vi "Image UDP Broadcast RT Driver VI.vi"(6 "Device Clock":string, 9 "Device Inputs FIFO":refnum<k33>, 10 "Device Outputs FIFO":refnum<k33>, 11 "Device Reference":T1 format="%.0x") -> ()   [LabVIEW 2012, in "Image UDP Broadcast Custom Device.lvlib"]
uses:
  Shared/Image UDP Broadcast Custom Device.lvlib
  <vilib>/NI Veristand/Custom Device API/Custom Device Item Ref.ctl
  <vilib>/NI Veristand/Custom Device API/Custom Device Channel Type.ctl
  <vilib>/vision/driver/IMAQdx.llb/IMAQdx Acquisition Mode.ctl
  <vilib>/NI Veristand/Custom Device API/Message Response (String).ctl
  <vilib>/NI Veristand/Custom Device API/Message Response (Byte Array).ctl
  <vilib>/vision/driver/IMAQdx.llb/IMAQdx Buffer Number Mode.ctl
  <vilib>/NI Veristand/Custom Device API/Custom Device API.lvlib
  <vilib>/NI Veristand/Custom Device Tools/Custom Device Utility Library/Custom Device Utility Library.lvlib
  <vilib>/vision/driver/NI_Vision_Acquisition_Software.lvlib
  <vilib>/vision/NI_Vision_Development_Module.lvlib
panel:
  in  "Initialization Status Notifier":refnum<notifier>
  in  "Status Notifier":refnum<notifier>
  # "Custom Device Template\nv1.0"
  # "Use this template as a starting point for creating a custom device code module. The input controls shown here are specially named controls that the system will use to provide the device loop with data. The controls are not required for the device loop to run. For instance, if the device doesn't produce any output data, then you don't need the Device Outputs FIFO control. If you do use these controls, however, they need to have these exact names to be functional."
  # "The optional status notifier element is used to notify the RT engine of the last state of the custom device, and to indicate the device has completed execution. If this control is not used, a default No Error value is returned to the system when the device finishes execution.\n\nNote: This error state is not checked until the system shuts down. Use an output status channel to send more immediate status values to the system."
  # "This optional input can be used to send the VeriStand Engine the final status of the custom device initalization process. If this control exists on the custom device front panel, the VeriStand Engine will wait for a status update before starting up. If the custom device reports an error, that will abort the execution of the current configuration in the VeriStand Engine.\n\nThis control can be deleted if the custom device does not need to send the initialization status update."
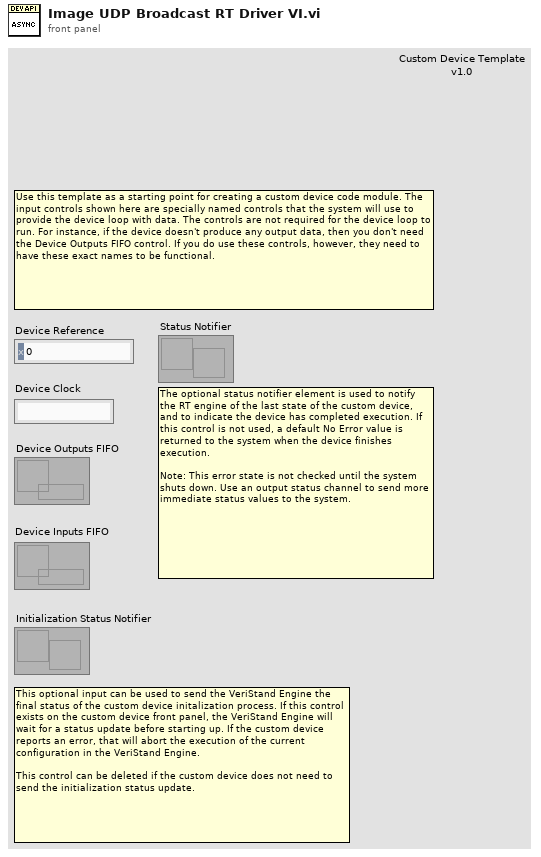
[diagram p1: front panel]
types:
  T1 = typedef "Custom Device API.lvlib/Custom Device Item Ref.ctl" = u64
  T2 = typedef "NI_Vision_Acquisition_Software.lvlib/IMAQdx Acquisition Mode.ctl" = enum32{"One Shot", "Continuous"}
  T3 = typedef "Image Type" = u32
  T4 = typedef "Custom Device API.lvlib/Custom Device Channel Type.ctl" = enum16{"Input", "Output"}
  T5 = typedef "Custom Device API.lvlib/Custom Device Engine Event Ref.ctl" = refnum<event-registration>
  T6 = typedef "Custom Device API.lvlib/Custom Device Item Info.ctl" = cluster{"Name":string, "Is Channel":bool, "GUID":string, "Is Waveform":bool}
  T7 = typedef "IMAQ Image.ctl" = refnum<image>
  T8 = typedef "IMAQdx.ctl" = refnum<k21>
  T9 = typedef "Custom Device API.lvlib/Message Response (String).ctl" = cluster{"Response":string, "Error":errorcluster}
  T10 = typedef "Custom Device API.lvlib/Message Response (Byte Array).ctl" = cluster{"Response":u8[], "Error":errorcluster}
  T11 = typedef "NI_Vision_Acquisition_Software.lvlib/IMAQdx Buffer Number Mode.ctl" = enum32{"Next", "Last", "Buffer Number"}
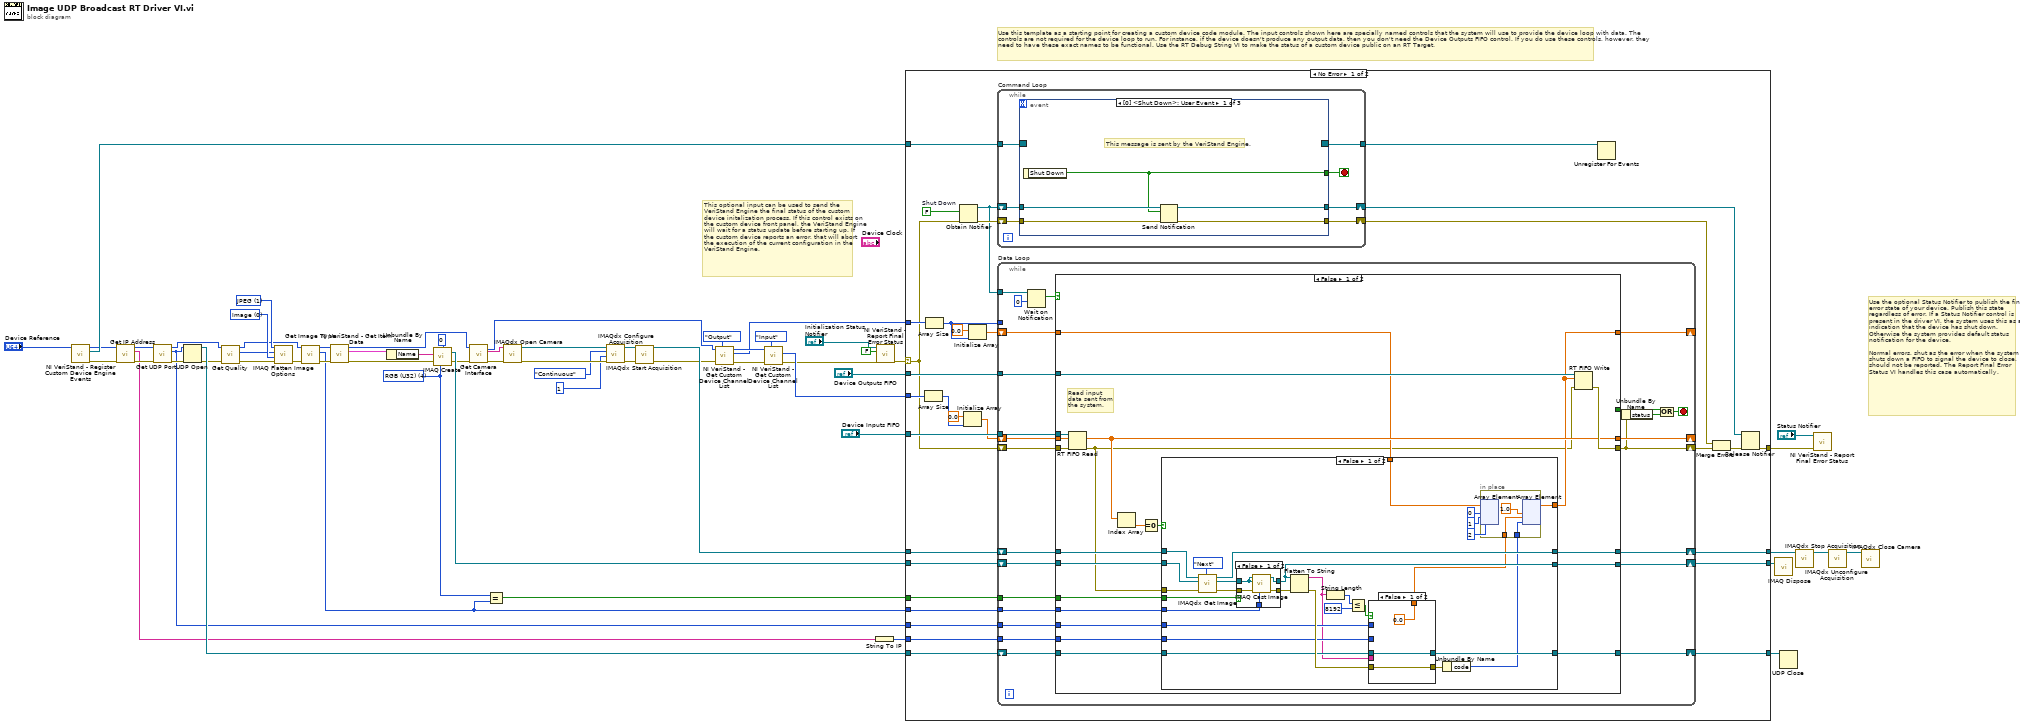
[diagram p0: block diagram]
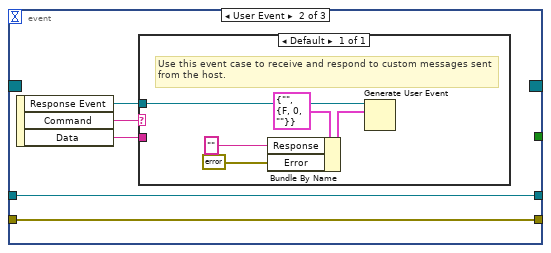
[diagram p2: hidden frame]
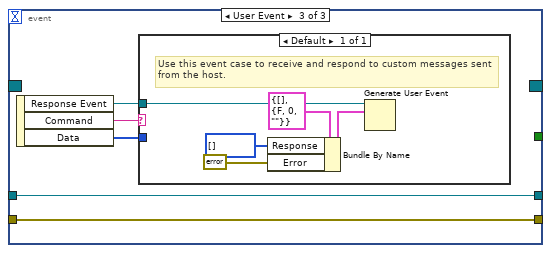
[diagram p3: hidden frame]
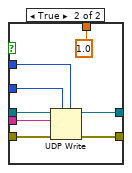
[diagram p5: hidden frame]
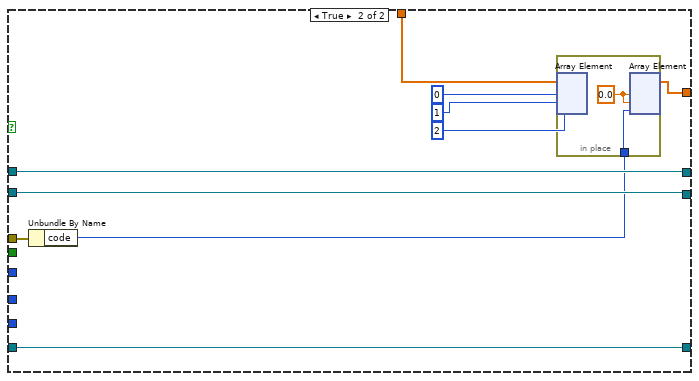
[diagram p6: hidden frame]
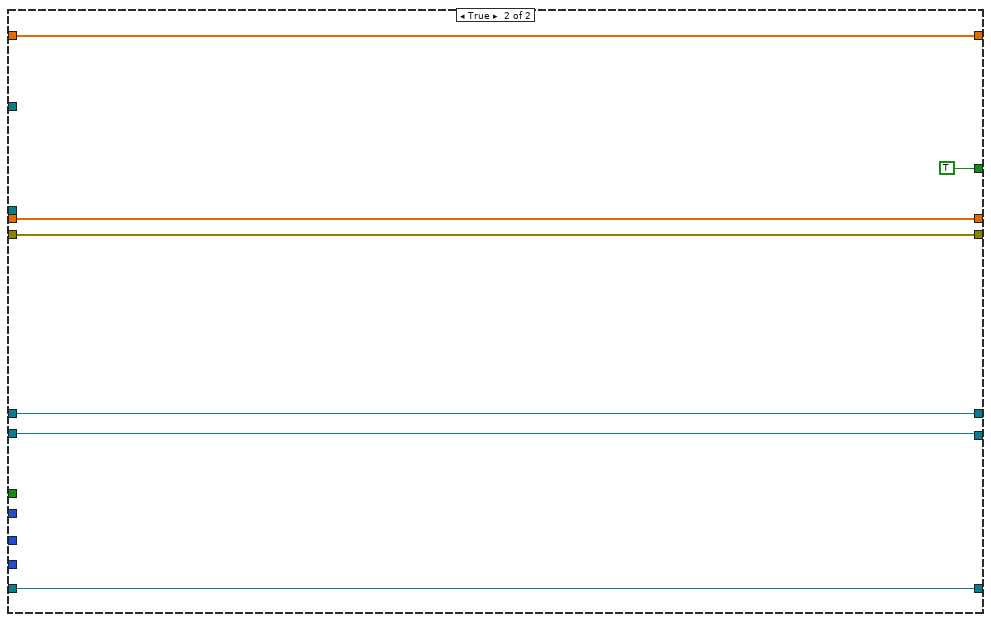
[diagram p7: hidden frame]
diagram:
  w3 = T3 4 items=["Grayscale (U8)", "Grayscale (I16)", "Grayscale (SGL)", "Complex (CSG)", "RGB (U32)", "HSL (U32)", "RGB (U64)", "Grayscale (U16)"] ("Image Type 2")
  w42 = 0 items=["Image", "Image and Vision Info", "Reference to Image"] ("Type of Flatten (Image and Vision Info)")
  w41 = 1 items=["None", "JPEG", "PACKED BINARY"] ("Compression (None)")
  # "This optional input can be used to send the VeriStand Engine the final status of the custom device initalization process. If this control exists on the custom device front panel, the VeriStand Engine will wait for a status update before starting up. If the custom device reports an error, that will abort the execution of the current configuration in the VeriStand Engine."
  # "Use the optional Status Notifier to publish the final error state of your device. Publish this state regardless of error. If a Status Notifier control is present in the driver VI, the system uses this as an indication that the device has shut down. Otherwise the system provides default status notification for the device.\n\nNormal errors, shut as the error when the system shuts down a FIFO to signal the device to close, should not be reported. The Report Final Error Status VI handles this case automatically."
  # "Use this template as a starting point for creating a custom device code module. The input controls shown here are specially named controls that the system will use to provide the device loop with data. The controls are not required for the device loop to run. For instance, if the device doesn't produce any output data, then you don't need the Device Outputs FIFO control. If you do use these controls, however, they need to have these exact names to be functional. Use the RT Debug String VI to make the status of a custom device public on an RT Target."
  n1 = call <vilib>:"NI VeriStand - Register Custom Device Engine Events.vi"("Device Ref in"="Device Reference") -> ("error out"=w12:errorcluster, "Custom Device Engine Event Ref"=w51:T5, "Device Ref out"=w14:T1)  [unwired: 8 in]
  n2 = call "Get IP Address.vi"("error in (no error)"=w12, "Dev Ref in"=w14) -> ("error out"=w11:errorcluster, "Value"=w10:string, "Dev Ref out"=w13:T1)  [unwired: 7 in]
  n3 = call "Get UDP Port.vi"("error in (no error)"=w11, "Dev Ref in"=w13) -> ("error out"=w44:errorcluster, "Value"=w26:u16, "Dev Ref out"=w27:T1)  [unwired: 7 in]
  n4 = UDP Open(8:w44, 11:w26) -> (port=w36:refnum<k16>, 0:w28:errorcluster)  [unwired: 3 in, 1 out]
  n5 = call "Get Quality.vi"("error in (no error)"=w28, "Dev Ref in"=w27) -> ("error out"=w40:errorcluster, "Value"=w30:i32, "Dev Ref out"=w38:T1)  [unwired: 7 in]
  n6 = call "IMAQ Flatten Image Options"("error in (no error)"=w40, "Type of Flatten (Image and Vision Info)"=w42, "Quality (750)"=w30, "Compression (None)"=w41) -> ("error out"=w39:errorcluster)  [unwired: 4 in, 3 out]
  n7 = call "Get Image Type.vi"("error in (no error)"=w39, "Dev Ref in"=w38) -> ("error out"=w7:errorcluster, "Value"=w2:T3, "Dev Ref out"=w9:T1)  [unwired: 7 in]
  n8 = call <vilib>:"NI VeriStand - Get Item Data.vi"("error in (no error)"=w7, "Item Ref in"=w9) -> ("error out"=w6:errorcluster, "Item Info"=w5:T6, "Item Ref out"=w8:T1)  [unwired: 6 in, 1 out]
  n9 = Unbundle By Name(w5) -> ("Name"=w4:string)
  n10 = call "IMAQ Create"("Border Size"=0, "Image Name"=w4, "Image Type"=w3, "error in (no error)"=w6) -> ("New Image"=w34:T7, "error out"=w29:errorcluster)  [unwired: 1 in]
  n11 = call "Get Camera Interface.vi"("error in (no error)"=w29, "Dev Ref in"=w8) -> ("error out"=w47:errorcluster, "Value"=w46:string, "Dev Ref out"=w24:T1)  [unwired: 7 in]
  n12 = Equal?(x=w3, y=w2) -> (x = y?=w1:bool)
  n13 = call <vilib>:"IMAQdx Open Camera.vi"("error in"=w47, "Session In"=w46) -> ("error out"=w45:errorcluster, "Session Out"=w43:T8)  [unwired: 8 in]
  n14 = call <vilib>:"IMAQdx Configure Acquisition.vi"("error in"=w45, "Number of Buffers"=u32 1, "Continuous?"=IMAQdx_Acquisition_Mode."Continuous", "Session In"=w43) -> ("error out"=w18:errorcluster, "Session Out"=w19:T8)  [unwired: 6 in]
  n15 = call <vilib>:"IMAQdx Start Acquisition.vi"("error in"=w18, "Session In"=w19) -> ("error out"=w25:errorcluster, "Session Out"=w35:T8)  [unwired: 8 in]
  n16 = call <vilib>:"NI VeriStand - Get Custom Device Channel List.vi"("Channel Type"=Custom_Device_Channel_Type."Output", "error in (no error)"=w25, "Device Ref in"=w24) -> ("error out"=w56:errorcluster, "Specified Channel Ref List"=w53:T1[], "Device Ref out"=w57:T1)  [unwired: 6 out]
  n17 = call <vilib>:"NI VeriStand - Get Custom Device Channel List.vi"("Channel Type"=Custom_Device_Channel_Type."Input", "error in (no error)"=w56, "Device Ref in"=w57) -> ("error out"=w23:errorcluster, "Specified Channel Ref List"=w54:T1[])  [unwired: 7 out]
  n18 = String To IP(1:w10) -> (0:w33:u32)
  n19 = call <vilib>:"NI VeriStand - Report Final Error Status.vi"("error in (no error)"=w23, "Filter FIFO & Shutdown Errors (T)"=FALSE ("Filter FIFO Errors (T)"), "Status Notifier"="Initialization Status Notifier") -> ("error out"=w49:errorcluster)  [unwired: 8 out]
  n20 = case shown="No Error" w49 {
    selector: w49 -> [w74 w241]
    tunnel: "Device Outputs FIFO" -> [w91 _]
    tunnel: "Device Inputs FIFO" -> [w90 _]
    tunnel: w54 -> [w84 _]
    tunnel: w53 -> [w83 _]
    tunnel: w51 -> [w81 _]
    tunnel: [w79 w241] -> w15
    tunnel: w36 -> [w71 w238]
    tunnel: w35 -> [w70 w239]
    tunnel: w34 -> [w69 w240]
    tunnel: w2 -> [w68 _]
    tunnel: w33 -> [w67 _]
    tunnel: w26 -> [w66 _]
    tunnel: [w65 w240] -> w32
    tunnel: [w64 w239] -> w22
    tunnel: [w63 w238] -> w31
    tunnel: w1 -> [w62 _]
    frame No Error {
      w80 = FALSE  # Shut Down
      n21 = Array Size(array=w84) -> (size(s)=w82:i32)
      n22 = Array Size(array=w83) -> (size(s)=w85:i32)
      n23 = Obtain Notifier(notification data type=w80, error in (no error)=w74) -> (notifier out=w77:refnum<notifier>, error out=w92:errorcluster)  [unwired: 2 in, 1 out]
      n24 = Initialize Array(0.0 ("element"), w82) -> (w86:dbl[])
      n25 = Initialize Array(0.0 ("element"), w85) -> (w87:dbl[])
      n26 = while "Command Loop" {
        tunnel: w81 -> [w99]
        tunnel: [w98] -> w78
        shift-right: [w95] -> w76
        shift-left: w77 -> [w96]
        shift-right: [w93] -> w72
        shift-left: w92 -> [w94]
        stop <- w97 stop-if-true
        n27 = event shown="[0] <Shut Down>: User Event" {
          selector: w99 -> [_ _ _]
          dyn-events: [_ _ _] -> w98
          timeout: _ -> [_ _ _]
          tunnel: [w102 _ _] -> w97
          tunnel: w96 -> [w103 w107 w117]
          tunnel: [w104 w107 w117] -> w95
          tunnel: w94 -> [w101 w105 w115]
          tunnel: [w100 w105 w115] -> w93
          event User Event {
            # "This message is sent by the VeriStand Engine."
            n28 = event-data() -> ("Shut Down"=w102:bool)  [unwired: 1 in]
            n29 = Send Notification(notification=w102, notifier=w103, error in (no error)=w101) -> (notifier out=w104:refnum<notifier>, error out=w100:errorcluster)
          }
          event User Event {
            n30 = event-data() -> ("Response Event"=w106:refnum<user-event>, "Command"=w109:string, "Data"=w108:string)  [unwired: 1 in]
            n31 = case shown="Default" w109 {
              tunnel: w108 -> [_]
              tunnel: w106 -> [w114]
              frame Default {
                # "Use this event case to receive and respond to custom messages sent from the host."
                n32 = Bundle By Name(cluster=T9 {"Response"="", "Error"={"status"=FALSE, "code"=0, "source"=""}} ("event data"), "Response"="", "Error"=errorcluster {"status"=FALSE, "code"=0, "source"=""}) -> (w112:T9)
                n33 = Generate User Event(user event=w114, event data cluster=w112) -> ()  [unwired: 1 in, 2 out]
              }
            }
          }
          event User Event {
            n34 = event-data() -> ("Response Event"=w116:refnum<user-event>, "Command"=w119:string, "Data"=w118:u8[])  [unwired: 1 in]
            n35 = case shown="Default" w119 {
              tunnel: w118 -> [_]
              tunnel: w116 -> [w124]
              frame Default {
                # "Use this event case to receive and respond to custom messages sent from the host."
                n36 = Bundle By Name(cluster=T10 {"Response"=[], "Error"={"status"=FALSE, "code"=0, "source"=""}} ("event data"), "Response"=u8[] [], "Error"=errorcluster {"status"=FALSE, "code"=0, "source"=""}) -> (w121:T10)
                n37 = Generate User Event(user event=w124, event data cluster=w121) -> ()  [unwired: 1 in, 2 out]
              }
            }
          }
        }
      }
      n38 = while "Data Loop" {
        shift-right: [w146] -> _
        shift-left: w86 -> [w147]
        shift-right: [w140] -> w75
        shift-left: w74 -> [w148]
        shift-right: [w144] -> _
        shift-left: w87 -> [w145]
        tunnel: w85 -> [_]
        tunnel: w91 -> [w143]
        tunnel: w90 -> [w142]
        tunnel: w77 -> [w139]
        tunnel: w68 -> [w132]
        shift-right: [w131] -> w64
        shift-left: w70 -> [w134]
        shift-right: [w126] -> w65
        shift-left: w69 -> [w133]
        tunnel: w67 -> [w129]
        tunnel: w66 -> [w128]
        shift-right: [w127] -> w63
        shift-left: w71 -> [w130]
        tunnel: w62 -> [w125]
        stop <- w135 stop-if-true
        n39 = Wait on Notification(notifier=w139, timeout in ms (-1)=0) -> (notification=w138:bool)  [unwired: 2 in, 3 out]
        n40 = case shown="False" w138 {
          tunnel: w148 -> [w169 w236]
          tunnel: w147 -> [w168 w237]
          tunnel: [w163 w237] -> w146
          tunnel: w145 -> [w151 w235]
          tunnel: [w161 w235] -> w144
          tunnel: w143 -> [w167 _]
          tunnel: w142 -> [w166 _]
          tunnel: [w165 w236] -> w140
          tunnel: [_ TRUE] -> w136
          tunnel: w134 -> [w160 w233]
          tunnel: w133 -> [w159 w232]
          tunnel: w132 -> [w158 _]
          tunnel: [w157 w233] -> w131
          tunnel: w130 -> [w156 w231]
          tunnel: w129 -> [w155 _]
          tunnel: w128 -> [w154 _]
          tunnel: [w153 w231] -> w127
          tunnel: [w152 w232] -> w126
          tunnel: w125 -> [w149 _]
          frame False {
            # "Read input data sent from the system."
            n41 = RT FIFO Read(0:w166, 1:w168, 3:w169) -> (9:w163:dbl[], 11:w150:errorcluster)  [unwired: 4 out]
            n42 = Index Array(array=w163) -> (element=w164:dbl)  [unwired: 1 in]
            n43 = Equal To 0?(x=w164) -> (x = 0?=w162:bool)
            n44 = case shown="False" w162 {
              tunnel: [w178 w222] -> w161
              tunnel: w150 -> [w171 w220]
              tunnel: w160 -> [w197 w228]
              tunnel: w159 -> [w196 w226]
              tunnel: w158 -> [w181 _]
              tunnel: [w192 w228] -> w157
              tunnel: w156 -> [w188 w227]
              tunnel: w155 -> [w187 _]
              tunnel: w154 -> [w185 _]
              tunnel: [w184 w227] -> w153
              tunnel: [w182 w226] -> w152
              tunnel: w151 -> [w179 w223]
              tunnel: w149 -> [w170 _]
              frame False {
                n45 = call <vilib>:"IMAQdx Get Image.vi"("Buffer Number Mode (Next)"=IMAQdx_Buffer_Number_Mode."Next", "error in"=w171, "Image In"=w196, "Session In"=w197) -> ("error out"=w195:errorcluster, "Image Out"=w194:T7, "Session Out"=w192:T8)  [unwired: 4 in, 1 out]
                n46 = case shown="False" w170 {
                  tunnel: w195 -> [w202 w203]
                  tunnel: w194 -> [w201 w204]
                  tunnel: [w200 w203] -> w193
                  tunnel: [w199 w204] -> w182
                  tunnel: w181 -> [w198 _]
                  frame False {
                    n47 = call "IMAQ Cast Image"("Image Type"=w198, "error in (no error)"=w202, "Image Dst"=w201, "Image Src"=w201) -> ("error out"=w200:errorcluster, "Image Dst Out"=w199:T7)  [unwired: 6 in]
                  }
                  frame True {
                  }
                }
                n48 = Flatten To String(anything=w182, error in (no error)=w193) -> (data string=w183:string, error out=w189:errorcluster)  [unwired: 2 in, 1 out]
                n49 = String Length(string=w183) -> (length=w191:i32)
                n50 = Less Or Equal?(x=w191, y=8192) -> (x <= y?=w186:bool)
                n51 = case shown="False" w186 {
                  tunnel: w189 -> [w209 w218]
                  tunnel: w188 -> [w210 w217]
                  tunnel: w187 -> [_ w211]
                  tunnel: w185 -> [_ w216]
                  tunnel: [w210 w215] -> w184
                  tunnel: w183 -> [_ w214]
                  tunnel: [w209 w213] -> w174
                  tunnel: [0.0 1.0] -> w177
                  frame False {
                  }
                  frame True {
                    n52 = UDP Write(address=w211, port or service name=w216, connection ID=w217, data in=w214, 8:w218) -> (error out=w213:errorcluster, 3:w215:refnum<k16>)  [unwired: 1 in]
                  }
                }
                n53 = Unbundle By Name(w174) -> ("code"=w172:i32)
                n54 = in-place {
                  in-place-border: w177 -> [w206]
                  in-place-border: w172 -> [w205]
                  n55 = in-place-array #1(w179, 0, 1, 2) -> ()  [unwired: 3 out]
                  n56 = in-place-array #1(1.0, w206, w205) -> (w178:dbl[])  [unwired: 3 out]
                }
              }
              frame True {
                n57 = Unbundle By Name(w220) -> ("code"=w219:i32)
                n58 = in-place {
                  in-place-border: w219 -> [w229]
                  w230 = 0.0
                  n59 = in-place-array #2(w223, 0, 1, 2) -> ()  [unwired: 3 out]
                  n60 = in-place-array #2(w230, w230, w229) -> (w222:dbl[])  [unwired: 3 out]
                }
              }
            }
            n61 = RT FIFO Write(0:w167, 1:w161, 3:w150) -> (11:w165:errorcluster)  [unwired: 1 in, 4 out]
          }
          frame True {
          }
        }
        n62 = Unbundle By Name(w140) -> ("status"=w137:bool)
        n63 = Compound Arithmetic op=OR(w136, w137) -> (w135:bool)
      }
      n64 = Unregister For Events(event registration refnum=w78) -> ()  [unwired: 1 in, 1 out]
      n65 = Merge Errors(w72, w75) -> (w73:errorcluster)
      n66 = Release Notifier(notifier=w76, error in (no error)=w73) -> (error out=w79:errorcluster)  [unwired: 1 in, 2 out]
    }
    frame Error {
    }
  }
  n67 = call "IMAQ Dispose"("Image"=w32) -> ()  [unwired: 5 in, 1 out]
  n68 = UDP Close(connection ID=w31) -> ()  [unwired: 1 in, 2 out]
  n69 = call <vilib>:"IMAQdx Stop Acquisition.vi"("Session In"=w22) -> ("Session Out"=w21:T8)  [unwired: 9 in, 1 out]
  n70 = call <vilib>:"NI VeriStand - Report Final Error Status.vi"("error in (no error)"=w15, "Status Notifier"="Status Notifier") -> ()  [unwired: 1 in, 9 out]
  n71 = call <vilib>:"IMAQdx Unconfigure Acquisition.vi"("Session In"=w21) -> ("Session Out"=w20:T8)  [unwired: 9 in, 1 out]
  n72 = call <vilib>:"IMAQdx Close Camera.vi"("Session In"=w20) -> ()  [unwired: 10 in, 1 out]
